vi "WriteEventLog.vi"(10 "LogText":string, 11 "EventLog":string) -> (3 "EventLogOut":string)   [LabVIEW 2019]
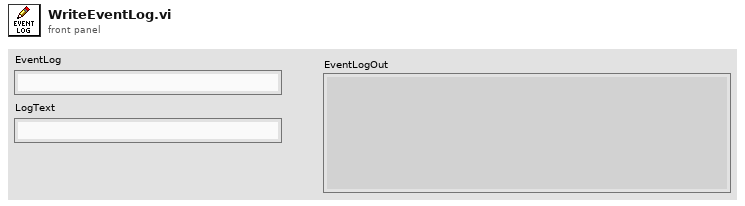
[diagram p1: front panel]
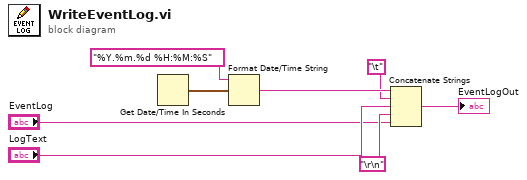
[diagram p0: block diagram]
diagram:
  n1 = Get Date/Time In Seconds() -> (seconds since 1Jan1904=w7:timestamp)
  n2 = Format Date/Time String(time format string (%c)="%Y.%m.%d %H:%M:%S", seconds (now)=w7) -> (date/time string=w5:string)  [unwired: 1 in]
  n3 = Concatenate Strings(w5, "\t", "LogText", "\r\n", "EventLog") -> (→"EventLogOut":string)
